vi "Cfg(VISA Cfg）.vi"(7 "R/W":enum16{"Read", "Write"}(ring), 8 "error in (no error)":errorcluster caption="错误输入（无错误）", 10 "串口配置":T1={"COM"="", "baud rate (9600)"=9600, "data bits (8)"=8, "parity (0:none)"=enum."None", "stop bits (10: 1 bit)"=10} {"stop bits (10: 1 bit)" items=["1.0"=10, "1.5"=15, "2.0"=20]; "data bits (8)" min=5 max=8 step=1}) -> (0 "error out":errorcluster caption="错误输出", 2 "串口配置":T1={"COM"="", "baud rate (9600)"=9600, "data bits (8)"=8, "parity (0:none)"=enum."None", "stop bits (10: 1 bit)"=10} {"stop bits (10: 1 bit)" items=["1.0"=10, "1.5"=15, "2.0"=20]; "data bits (8)" min=5 max=8 step=1})   [LabVIEW 2020, in "人体健康监测系统.lvclass"]
uses:
  <vilib>/Utility/config.llb/Read Key (String).vi
  <vilib>/Utility/config.llb/Write Key (String).vi
  <vilib>/Utility/config.llb/NI_LVConfig.lvlib
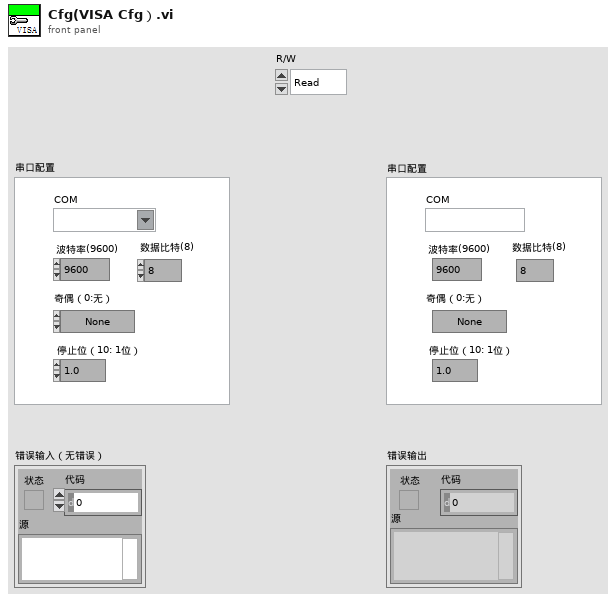
[diagram p1: front panel]
types:
  T1 = typedef "人体健康监测系统.lvclass/串口配置.ctl" = cluster{"COM":refnum<visa-resource-name>, "baud rate (9600)":u32, "data bits (8)":u16, "parity (0:none)":enum16{"None", "Odd", "Even", "Mark", "Space"}, "stop bits (10: 1 bit)":u16}
  T2 = typedef "NI_LVConfig.lvlib/Config Data RefNum.ctl" = refnum<k1>
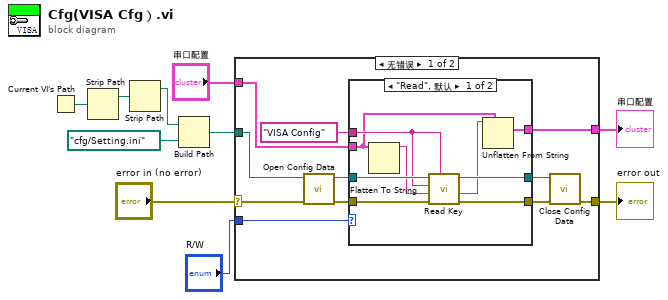
[diagram p0: block diagram]
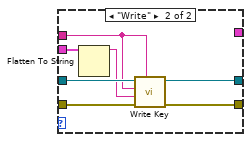
[diagram p2: hidden frame]
diagram:
  n1 = Current VI's Path() -> (path=w8:path)
  n2 = Strip Path(path=w8) -> (stripped path=w2:path)  [unwired: 1 out]
  n3 = Strip Path(path=w2) -> (stripped path=w1:path)  [unwired: 1 out]
  n4 = Build Path(base path=w1, name or relative path=path "cfg/Setting.ini" ("名称或相对路径")) -> (appended path=w6:path)
  n5 = case shown="无错误" "error in (no error)" {
    selector: "error in (no error)" -> [w20 w38]
    tunnel: [w11 w38] -> w9
    tunnel: w6 -> [w21 _]
    tunnel: "R/W" -> [w19 _]
    tunnel: "串口配置" -> [w16 _]
    tunnel: [w14 _] -> w3
    frame No Error {
      n6 = call <vilib>:"Open Config Data.vi"("error in (no error)"=w20, "configuration file path"=w21) -> ("error out"=w17:errorcluster, "refnum"=w18:T2)  [unwired: 7 in, 1 out]
      n7 = case shown="\"Read\", 默认" w19 {
        tunnel: w18 -> [w30 w37]
        tunnel: w17 -> [w29 w36]
        tunnel: w16 -> [w23 w35]
        tunnel: [w27 w33] -> w12
        tunnel: [w28 w32] -> w13
        tunnel: "VISA Config" ("section") -> [w26 w31]
        tunnel: [w24 _] -> w14
        frame "Read", Default {
          n8 = Flatten To String(anything=w23) -> (data string=w22:string)  [unwired: 3 in, 2 out]
          n9 = call-poly <vilib>:"Read Key.vi"("section"=w26, "error in (no error)"=w29, "default value"=w22, "key"=w26, "refnum"=w30) -> ("error out"=w27:errorcluster, "value"=w25:string, "refnum out"=w28:T2)  [unwired: 3 in, 1 out]
          n10 = Unflatten From String(type=w23, binary string=w25) -> (value=w24:T1)  [unwired: 3 in, 2 out]
        }
        frame "Write" {
          n11 = Flatten To String(anything=w35) -> (data string=w34:string)  [unwired: 3 in, 2 out]
          n12 = call-poly <vilib>:"Write Key.vi"("section"=w31, "error in (no error)"=w36, "value"=w34, "key"=w31, "refnum"=w37) -> ("error out"=w33:errorcluster, "refnum out"=w32:T2)  [unwired: 4 in, 1 out]
        }
      }
      n13 = call <vilib>:"Close Config Data.vi"("error in (no error)"=w12, "refnum"=w13) -> ("error out"=w11:errorcluster)  [unwired: 8 in, 1 out]
    }
    frame Error {
    }
  }
  "error out" <- w9
  "串口配置" <- w3
